vi "Write Status.vi"(8 "error in (no error)":errorcluster, 10 "Status":string, 11 "Send-status in":refnum<class "Send-status.lvclass">) -> (0 "error out":errorcluster, 3 "Send-status out":refnum<class "Send-status.lvclass">)   [LabVIEW 2013, in "SLMAPI.lvlib" / "Send-status.lvclass"]
uses:
  Send-status.lvclass
  Send-status.lvclass/Send-status.ctl
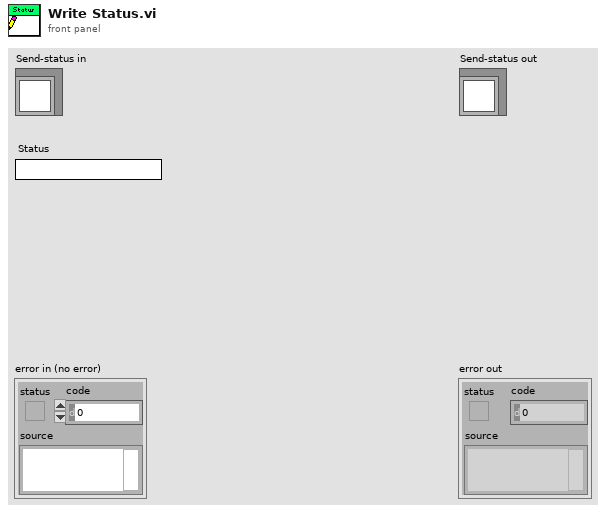
[diagram p1: front panel]
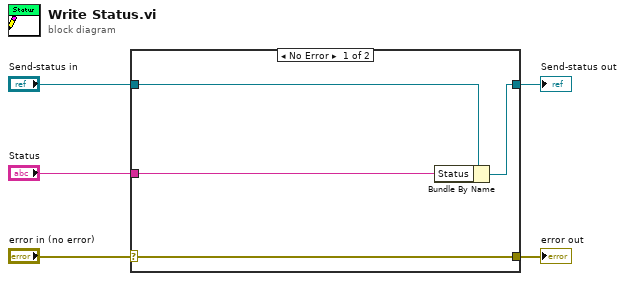
[diagram p0: block diagram]
diagram:
  n1 = case shown="No Error" "error in (no error)" {
    selector: "error in (no error)" -> [w9 w10]
    tunnel: [w9 w10] -> w4
    tunnel: [w7 w11] -> w2
    tunnel: "Send-status in" -> [w8 w11]
    tunnel: "Status" -> [w6 _]
    frame No Error {
      n2 = Bundle By Name(cluster=w8, "Status"=w6) -> (w7:refnum<class "Send-status.lvclass">)
    }
    frame Error {
    }
  }
  "error out" <- w4
  "Send-status out" <- w2
